vi "getGeneralLocation.vi"(8 "error in (no error)":errorcluster, 11 "PassBuoys in":refnum<class "PassBuoys.lvclass">) -> (0 "error out":errorcluster, 2 "General Location":T1 {"North" format="%#_10f"; "East" format="%#_8f"}, 3 "PassBuoys out":refnum<class "PassBuoys.lvclass">)   [LabVIEW 2011, in "PassBuoys.lvclass"]
uses:
  PassBuoys.lvclass
  2 Typedefs/UTM Location.ctl
  PassBuoys.lvclass/PassBuoys.ctl
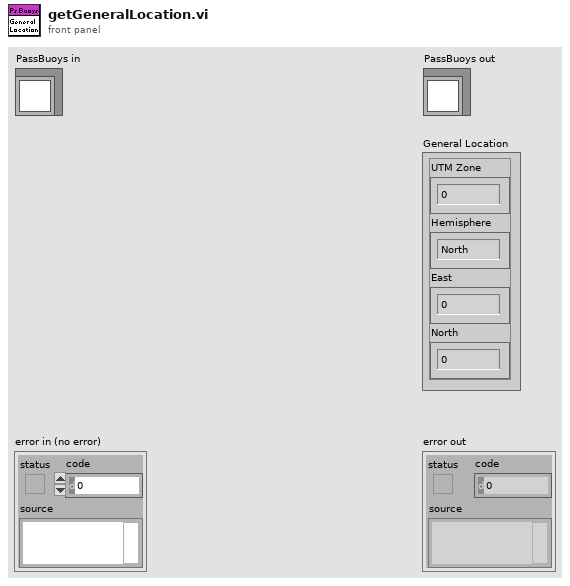
[diagram p1: front panel]
types:
  T1 = typedef "UTM Location.ctl" = cluster{"UTM Zone":dbl, "Hemisphere":enum16{"North", "South"}, "East":dbl, "North":dbl}
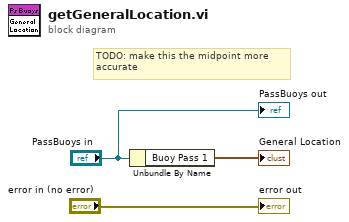
[diagram p0: block diagram]
diagram:
  # "TODO: make this the midpoint more\naccurate"
  n1 = Unbundle By Name("PassBuoys in") -> ("Buoy Pass 1"=→"General Location":T1)
  "error out" <- "error in (no error)"
  "PassBuoys out" <- "PassBuoys in"
